vi "LOOP_pp3c_updateSideState.vi"(8 "error in (no error)":errorcluster, 9 "log queue in":refnum<queue>, 10 "Daq config In":T1={"Sound AO"="Dev6/ao0", "Shock intesity AO"="Dev6/ao1", "Code_LED DO"="Dev6/port1:2", "Switch DI"="Dev6/port1/line0", "Webcam"="cam9", "Sound AO task"="", "Sound card task"=0, "Shock intensity AO task"="", "Code_LED DO task"="", "Switch DI task"="", "AO <=> Sound card"=FALSE, "Sound card"=0, "sample rate"=100000.0, "Variable shock"=TRUE, "Webcam on"=FALSE, "Waveform memo"={"t0"=timestamp(0 s since 1904-01-01), "dt"=1.0, "Y"=[]}, "Tone trigger"="PFI1", "Master-9 DO"="", "Master-9 DO task"="Dev6/port0/line5:7", "Master-9 on"=TRUE} {"sample rate" min=8000.0; "Sound card task" format="%.0x"}, 11 "State In":T4={"Curr  tr"=0, "Curr (ms)"=0, "Cum (ms)"=0, "Run loop diff"=0, "Tone countdown (ms)"=0, "Countdown (ms)"=0, "Curr State"=enum."0 NULL", "Prev State"=enum."1 Habituation", "Rw"=FALSE, "Sw"=FALSE, "Tone\nGate"=FALSE, "Punish"=FALSE, "Current DAQ DO Int"=0, "Current Loaded Trial"={"Trial Type Number"=1, "Trial Type"=enum."GO", "Trial Weight"=100, "Shock (mA)"=0.3, "Duration (ms)"=0.25, "Sound Type"=enum."04 FM Sweep", "Stim P1"=4000.0, "Stim P2"=0.0, "Stim P3"=0.0, "Stim P4"=2000.0, "DAQ Amplitude (V)"=0.25}, "Total trials memo"=0, "State start cum memo (ms)"=0, "Last dur jump time memo (ms)"=0, "Last dur shock time memo (ms)"=0, "Tone repeat memo (ms)"=0, "Webcam on"=FALSE, "Webcam recording"=FALSE, "State update flag"=FALSE, "Last loaded shock voltage"=0.0, "Vid upd"=enum."0", "First time tone"=FALSE} {"Current DAQ DO Int" format="%016b"; "Current Loaded Trial"."DAQ Amplitude (V)" min=0.0 max=5.0 format="%_4g"; "Current Loaded Trial"."Shock (mA)" min=-1.0 max=5.0; "Current Loaded Trial"."Trial Weight" step=1; "Current Loaded Trial"."Duration (ms)" min=0.0 max=1.0; "Current Loaded Trial"."Trial Type Number" min=1 max=256 step=1}) -> (0 "error out":errorcluster, 1 "log queue out":refnum<queue>, 3 "State Out":T4={"Curr  tr"=0, "Curr (ms)"=0, "Cum (ms)"=0, "Run loop diff"=0, "Tone countdown (ms)"=0, "Countdown (ms)"=0, "Curr State"=enum."0 NULL", "Prev State"=enum."1 Habituation", "Rw"=FALSE, "Sw"=FALSE, "Tone\nGate"=FALSE, "Punish"=FALSE, "Current DAQ DO Int"=0, "Current Loaded Trial"={"Trial Type Number"=1, "Trial Type"=enum."GO", "Trial Weight"=100, "Shock (mA)"=0.3, "Duration (ms)"=0.25, "Sound Type"=enum."04 FM Sweep", "Stim P1"=4000.0, "Stim P2"=0.0, "Stim P3"=0.0, "Stim P4"=2000.0, "DAQ Amplitude (V)"=0.25}, "Total trials memo"=0, "State start cum memo (ms)"=0, "Last dur jump time memo (ms)"=0, "Last dur shock time memo (ms)"=0, "Tone repeat memo (ms)"=0, "Webcam on"=FALSE, "Webcam recording"=FALSE, "State update flag"=FALSE, "Last loaded shock voltage"=0.0, "Vid upd"=enum."0", "First time tone"=FALSE} {"Current DAQ DO Int" format="%016b"; "Current Loaded Trial"."DAQ Amplitude (V)" min=0.0 max=5.0 format="%_4g"; "Current Loaded Trial"."Shock (mA)" min=-1.0 max=5.0; "Current Loaded Trial"."Trial Weight" step=1; "Current Loaded Trial"."Duration (ms)" min=0.0 max=1.0; "Current Loaded Trial"."Trial Type Number" min=1 max=256 step=1}, 4 "State timeout":bool, 6 "Side change":bool)   [LabVIEW 2013]
uses:
  CTL_pp3c_LoopState.ctl
  pp3_CTL_BehavioralState.ctl
  pp3_CTL_Trial.ctl
  pp3_CTL_TrialType.ctl
  labolabo2/waveforms/WFTypes.ctl
  CTL_pp3c_DaqStatus.ctl
  <vilib>/userdefined/High Color/IMAQdx.ctl
  <vilib>/sound2/lvsound2.llb/Sound Output Task ID.ctl
  <vilib>/DAQmx/read.llb/DAQmx Read (Digital Bool 1Line 1Point).vi
  <vilib>/DAQmx/miscellaneous.llb/DAQmx Fill In Error Info.vi
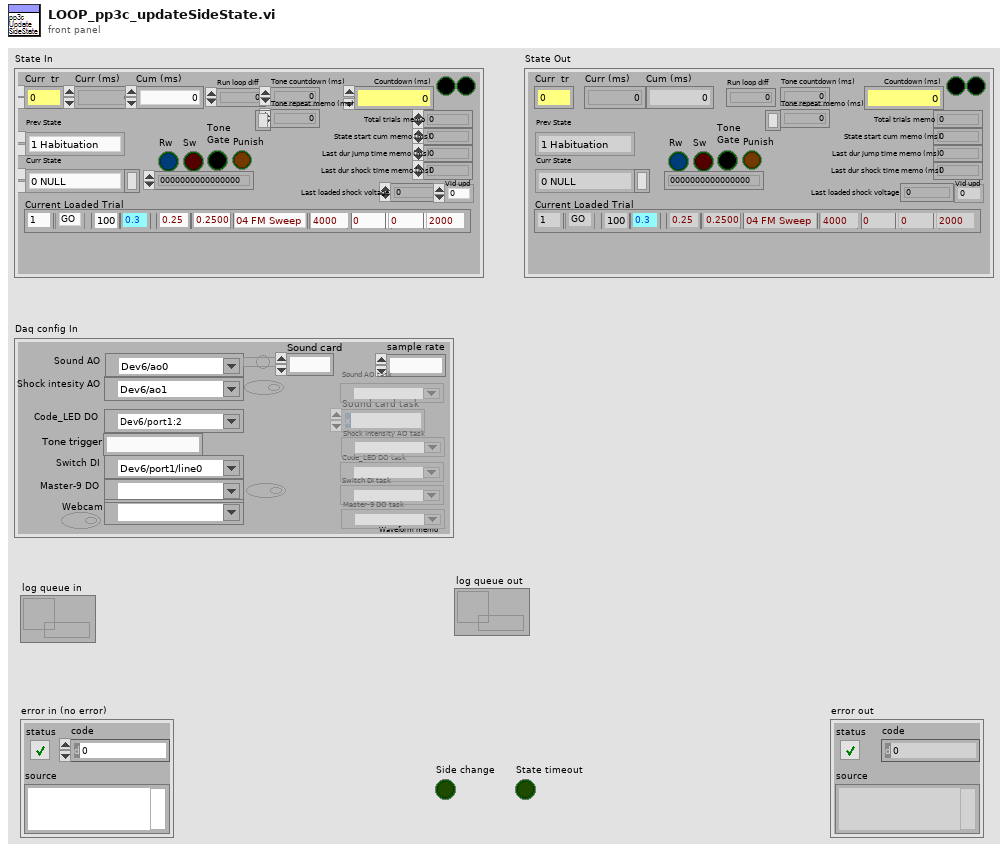
[diagram p1: front panel]
types:
  T1 = typedef "CTL_pp3c_DaqStatus.ctl" = cluster{"Sound AO":tag, "Shock intesity AO":tag, "Code_LED DO":tag, "Switch DI":tag, "Webcam":T2, "Sound AO task":refnum<k21>, "Sound card task":T3, "Shock intensity AO task":refnum<k21>, "Code_LED DO task":refnum<k21>, "Switch DI task":refnum<k21>, "AO <=> Sound card":bool, "Sound card":u32, "sample rate":dbl, "Variable shock":bool, "Webcam on":bool, "Waveform memo":waveform(dbl), "Tone trigger":string, "Master-9 DO":tag, "Master-9 DO task":refnum<k21>, "Master-9 on":bool}
  T2 = typedef "IMAQdx.ctl" = refnum<k21>
  T3 = typedef "Sound Output Task ID.ctl" = u32
  T4 = typedef "CTL_pp3c_LoopState.ctl" = cluster{"Curr  tr":u16, "Curr (ms)":u32, "Cum (ms)":u64, "Run loop diff":i64, "Tone countdown (ms)":i64, "Countdown (ms)":i64, "Curr State":T5, "Prev State":T5, "Rw":bool, "Sw":bool, "Tone\nGate":bool, "Punish":bool, "Current DAQ DO Int":u16, "Current Loaded Trial":T6, "Total trials memo":i64, "State start cum memo (ms)":i64, "Last dur jump time memo (ms)":i64, "Last dur shock time memo (ms)":i64, "Tone repeat memo (ms)":i64, "Webcam on":bool, "Webcam recording":bool, "State update flag":bool, "Last loaded shock voltage":dbl, "Vid upd":enum16{"0", "1", "2", "3", "4", "5", "6", "7", "8", "9"}, "First time tone":bool}
  T5 = typedef "pp3_CTL_BehavioralState.ctl" = enum8{"0 NULL", "1 Habituation", "2 (Load Trial)", "3 Stay Period", "4 Load Audio/Click Delay", "5 GO Trial", "6 GO Jumped", "7 GO Timeout", "8 NOGO Trial", "9 NOGO Jumped", "10 NOGO Timeout", "11 TEST Trial", "12 TEST Jumped", "13 TEST Timeout", "14 Intertrial Interval", "15 Done"}
  T6 = typedef "pp3_CTL_Trial.ctl" = cluster{"Trial Type Number":i16, "Trial Type":T7, "Trial Weight":u32, "Shock (mA)":dbl, "Duration (ms)":dbl, "Sound Type":T8, "Stim P1":dbl, "Stim P2":dbl, "Stim P3":dbl, "Stim P4":dbl, "DAQ Amplitude (V)":dbl}
  T7 = typedef "pp3_CTL_TrialType.ctl" = enum16{"OFF", "GO", "NOGO", "TEST"}
  T8 = typedef "WFTypes.ctl" = enum16{"00 NULL", "01 DC", "02 Noise", "03 Pure Tone", "04 FM Sweep"}
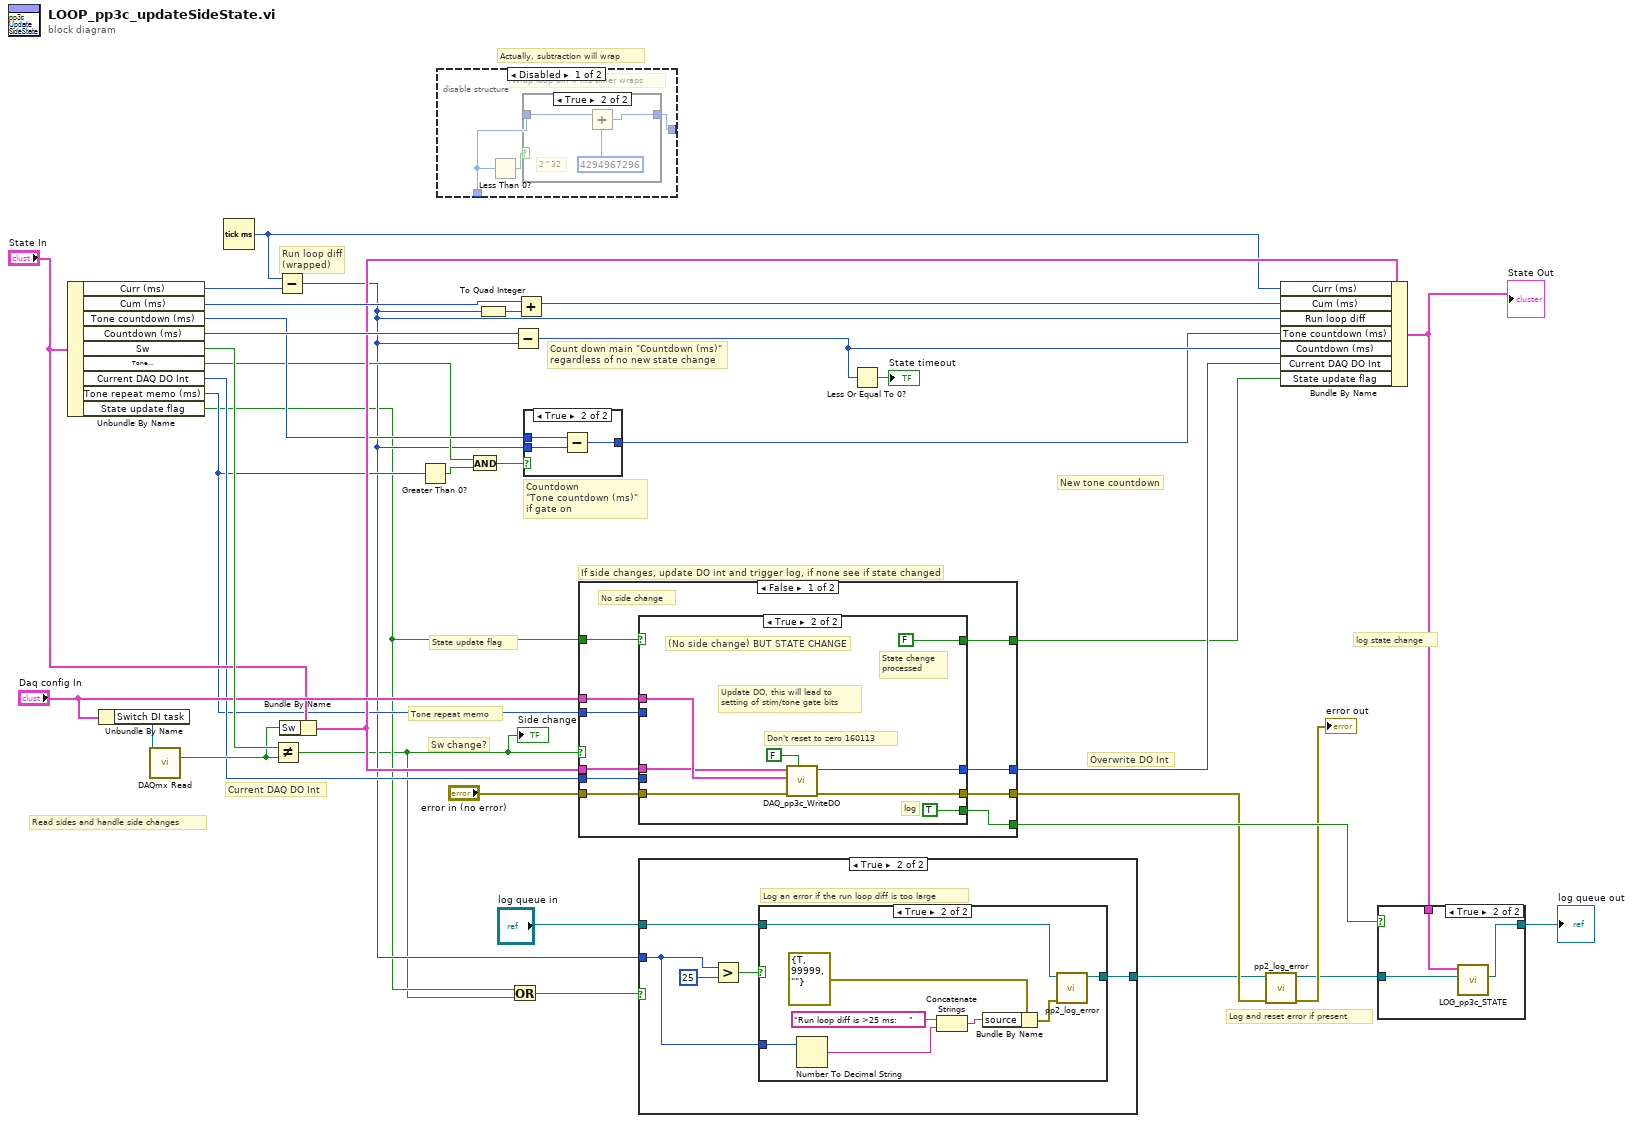
[diagram p0: block diagram]
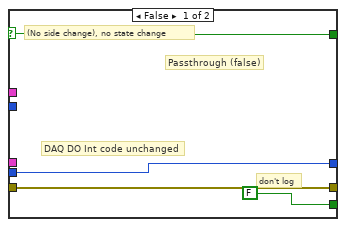
[diagram p8: hidden frame]
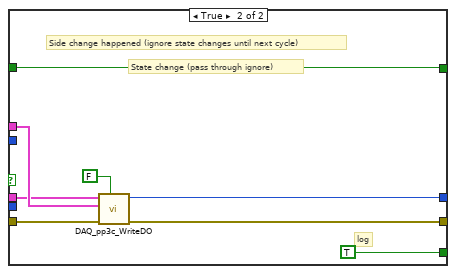
[diagram p9: hidden frame]
diagram:
  # "Overwrite DO Int"
  # "Actually, subtraction will wrap"
  # "Log and reset error if present"
  # "New tone countdown"
  # "Countdown \n\"Tone countdown (ms)\" \nif gate on"
  # "Tone repeat memo"
  # "Sw change?"
  # "Current DAQ DO Int"
  # "Count down main \"Countdown (ms)\" \nregardless of no new state change"
  # "State update flag"
  # "Run loop diff\n(wrapped)"
  # "If side changes, update DO int and trigger log, if none see if state changed"
  # "Read sides and handle side changes"
  # "log state change"
  n1 = Unbundle By Name("State In") -> ("Curr (ms)"=w36:u32, "Cum (ms)"=w35:u64, "Tone countdown (ms)"=w21:i64, "Countdown (ms)"=w33:i64, "Sw"=w31:bool, "Tone\nGate"=w12:bool, "Current DAQ DO Int"=w14:u16, "Tone repeat memo (ms)"=w10:i64, "State update flag"=w3:bool)
  n2 = Unbundle By Name("Daq config In") -> ("Switch DI task"=w32:refnum<k21>)
  n3 = call-poly <vilib>:"DAQmx Read.vi"("task/channels in"=w32) -> ("data"=w20:bool)  [unwired: 12 in, 2 out]
  n4 = Tick Count (ms)() -> (millisecond timer value=w19:u32)
  n5 = Not Equal?(x=w31, y=w20) -> (x != y?=w2:bool)
  "Side change" <- w2
  n6 = Subtract(x=w19, y=w36) -> (x-y=w9:u32)
  n7 = Bundle By Name(cluster="State In", "Sw"=w20) -> (w22:T4)
  n8 = Greater Than 0?(x=w10) -> (x > 0?=w11:bool)
  n9 = disable-structure shown="Disabled" {
    disable-tunnel: [w38 _] -> _
    disable-tunnel: [w37 _] -> _
    frame Disabled {
      # "Wrap loop diff if ms timer wraps"
      n10 = Less Than 0?(x=w38) -> (x < 0?=w39:bool)
      n11 = case shown="True" w39 {
        tunnel: [w40 w42] -> w38
        tunnel: [w40 w43] -> w37
        frame False {
        }
        frame True {
          # "2^32"
          n12 = Add(x=w42, y=i64 4294967296) -> (x+y=w43:i64)
        }
      }
    }
    frame Enabled {
    }
  }
  n13 = And(x=w12, y=w11) -> (x .and. y?=w13:bool)
  n14 = To Quad Integer(1:w9) -> (0:w18:i64)
  n15 = Or(x=w3, y=w2) -> (x .or. y?=w4:bool)
  n16 = Subtract(x=w33, y=w9) -> (x-y=w30:i64)
  n17 = Add(x=w35, y=w18) -> (x+y=w34:u64)
  n18 = case shown="True" w13 {
    tunnel: [w44 w45] -> w1
    tunnel: w21 -> [w44 w47]
    tunnel: w9 -> [_ w46]
    frame False {
      # "Passthrough if\ntone gate off"
    }
    frame True {
      n19 = Subtract(x=w47, y=w46) -> (x-y=w45:i64)
    }
  }
  n20 = case shown="False" w2 {
    tunnel: "Daq config In" -> [w51 w76]
    tunnel: [w56 w70] -> w23
    tunnel: w14 -> [w57 _]
    tunnel: "error in (no error)" -> [w50 w75]
    tunnel: [w54 w74] -> w16
    tunnel: [w55 TRUE] -> w26
    tunnel: w10 -> [w49 _]
    tunnel: w3 -> [w53 w73]
    tunnel: w22 -> [w52 w71]
    tunnel: [w48 w73] -> w17
    frame False {
      # "No side change"
      n21 = case shown="True" w53 {
        selector: w53 -> [w59 _]
        tunnel: w57 -> [w58 _]
        tunnel: [w58 w63] -> w56
        tunnel: w51 -> [_ w69]
        tunnel: [FALSE TRUE] -> w55
        tunnel: w50 -> [w60 w67]
        tunnel: [w60 w66] -> w54
        tunnel: w52 -> [_ w62]
        tunnel: w49 -> [_ _]
        tunnel: [w59 FALSE] -> w48
        frame False {
          # "Passthrough (false)"
          # "don't log"
          # "DAQ DO Int code unchanged"
          # "(No side change), no state change"
        }
        frame True {
          # "Don't reset to zero 160113"
          # "State change\nprocessed"
          # "log"
          # "Update DO, this will lead to\nsetting of stim/tone gate bits"
          # "(No side change) BUT STATE CHANGE"
          n22 = call "DAQ_pp3c_WriteDO.vi"("Reset to zero"=FALSE, "error in (no error)"=w67, "Daq config"=w69, "State In"=w62) -> ("error out"=w66:errorcluster, "DAQ Output Int"=w63:u16)  [unwired: 6 in]
        }
      }
    }
    frame True {
      # "State change (pass through ignore)"
      # "log"
      # "Side change happened (ignore state changes until next cycle)"
      n23 = call "DAQ_pp3c_WriteDO.vi"("Reset to zero"=FALSE, "error in (no error)"=w75, "Daq config"=w76, "State In"=w71) -> ("error out"=w74:errorcluster, "DAQ Output Int"=w70:u16)  [unwired: 6 in]
    }
  }
  n24 = case shown="True" w4 {
    tunnel: w9 -> [_ w81]
    tunnel: "log queue in" -> [w78 w80]
    tunnel: [w78 w79] -> w7
    frame False {
    }
    frame True {
      # "Log an error if the run loop diff is too large"
      n25 = Greater?(x=w81, y=u32 25) -> (0:w82:bool)
      n26 = case shown="True" w82 {
        tunnel: w81 -> [_ w91]
        tunnel: w80 -> [w84 w86]
        tunnel: [w84 w85] -> w79
        frame False {
        }
        frame True {
          n27 = Number To Decimal String(number=w91) -> (decimal integer string=w88:string)  [unwired: 1 in]
          n28 = Concatenate Strings("Run loop diff is >25 ms:    " ("string"), w88) -> (w90:string)
          n29 = Bundle By Name(cluster=errorcluster {"status"=TRUE, "code"=99999, "source"=""} ("error in (no error)"), "source"=w90) -> (w87:errorcluster)
          n30 = call "pp2_log_error.vi"("error in (no error)"=w87, "queue in"=w86) -> ("queue out"=w85:refnum<queue>)  [unwired: 6 in, 1 out]
        }
      }
    }
  }
  n31 = Less Or Equal To 0?(x=w30) -> (x <= 0?=→"State timeout":bool)
  n32 = call "pp2_log_error.vi"("error in (no error)"=w16, "queue in"=w7) -> ("error out"=→"error out":errorcluster, "queue out"=w6:refnum<queue>)  [unwired: 6 in]
  n33 = Bundle By Name(cluster=w22, "Curr (ms)"=w19, "Cum (ms)"=w34, "Run loop diff"=w9, "Tone countdown (ms)"=w1, "Countdown (ms)"=w30, "Current DAQ DO Int"=w23, "State update flag"=w17) -> (w25:T4)
  "State Out" <- w25
  n34 = case shown="True" w26 {
    tunnel: w25 -> [_ w96]
    tunnel: w6 -> [w93 w95]
    tunnel: [w93 w94] -> w5
    frame False {
    }
    frame True {
      n35 = call "LOG_pp3c_STATE.vi"("queue in"=w95, "State In"=w96) -> ("queue out"=w94:refnum<queue>)  [unwired: 9 in]
    }
  }
  "log queue out" <- w5
